vi "testReadStatusNotifier_tel.vi"(8 "error in (no error)":errorcluster) -> (0 "error out":errorcluster)   [LabVIEW 2018]
doc: "Test the readStatusNotifier.vi with tel selection."
uses:
  src/TcpServer/TcpServer.lvclass
  src/TcpServer/TcpServer.lvclass/TcpServer.ctl
  src/TcpServerBase/TcpServerBase.lvclass/TcpServerBase.ctl
  src/TcpServerTel/TcpServerTel.lvclass
  home/pcortes/github/ts_labview_tcp_json/src/TcpServerBase/TcpServerBase.lvclass
  <vilib>/addons/_JKI Toolkits/Caraya/classes/Assert/Assert Equal Type_Variant.vi
  <vilib>/addons/_JKI Toolkits/Caraya/classes/Test/Test.lvclass
  <vilib>/addons/_JKI Toolkits/Caraya/classes/Assert/Assert.lvclass
  src/TcpServerBase/TcpServerBase.lvclass
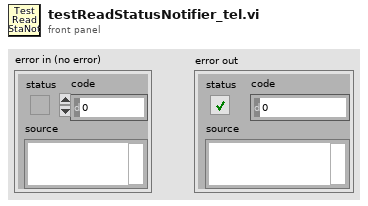
[diagram p1: front panel]
types:
  T1 = cluster{"connectionStatus":bool, "errorSource":string}
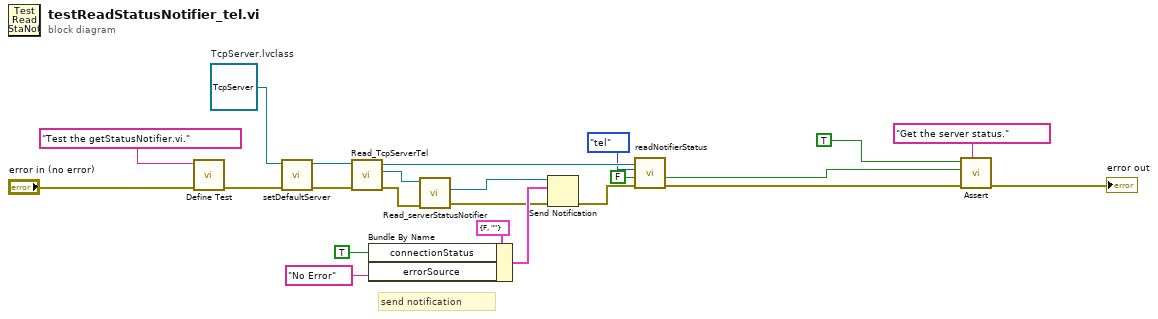
[diagram p0: block diagram]
diagram:
  w17 = refnum<class "TcpServer.lvclass"> refnum  # TcpServer.lvclass
  # "send notification"
  n1 = call <vilib>:"Define Test.vi"("error in (no error)"="error in (no error)", "Label (VI Title)"="Test the getStatusNotifier.vi.") -> ("error out"=w16:errorcluster)  [unwired: 9 in]
  n2 = call "setDefaultServer.vi"("error in (no error)"=w16, "TcpServer.lvclass"=w17) -> ("error out"=w15:errorcluster, "tcpServer out"=w14:refnum<class "TcpServer.lvclass">)  [unwired: 8 in]
  n3 = call "Read_TcpServerTel.vi"("error in (no error)"=w15, "TcpServer in"=w14) -> ("error out"=w13:errorcluster, "TcpServerTel.lvclass"=w12:refnum<class "TcpServerTel.lvclass">, "TcpServer out"=w4:refnum<class "TcpServer.lvclass">)  [unwired: 7 in]
  n4 = Bundle By Name(cluster=T1 {"connectionStatus"=FALSE, "errorSource"=""} ("notification"), "connectionStatus"=TRUE, "errorSource"="No Error" ("source")) -> (w7:T1)
  n5 = call "Read_serverStatusNotifier.vi"("error in (no error)"=w13, "TcpServerBase in"=w12) -> ("error out"=w6:errorcluster, "serverStatusNotifier"=w11:refnum<notifier>)  [unwired: 7 in, 1 out]
  n6 = Send Notification(notification=w7, notifier=w11, error in (no error)=w6) -> (error out=w5:errorcluster)  [unwired: 1 out]
  n7 = call "readNotifierStatus.vi"("error in (no error)"=w5, "notifierStatus"=FALSE ("notification in"), "serverSelection"=enum16{"cmd", "tel"}."tel", "TcpServer in"=w4) -> ("error out (no error)"=w18:errorcluster, "notifierStatus"=w19:bool)  [unwired: 5 in, 1 out]
  n8 = call-poly <vilib>:"Assert.vi"("Label"="Get the server status.", "error in (no error)"=w18, "Y"=w19, "X"=TRUE) -> ("error out"=→"error out":errorcluster)  [unwired: 7 in]
